vi "Clousure.vi"(8 "error in (no error)":errorcluster, 11 "CreatorA":refnum<class "CreatorA.lvclass">) -> (0 "error out":errorcluster, 3 "CreatorA":refnum<class "CreatorA.lvclass">)   [LabVIEW 2020, in "FactoryMethod.lvlib" / "FactoryMethodLazyEvaluation.lvlib" / "CreatorA.lvclass"]
uses:
  CreatorA.lvclass
  Creator/Creator.lvclass
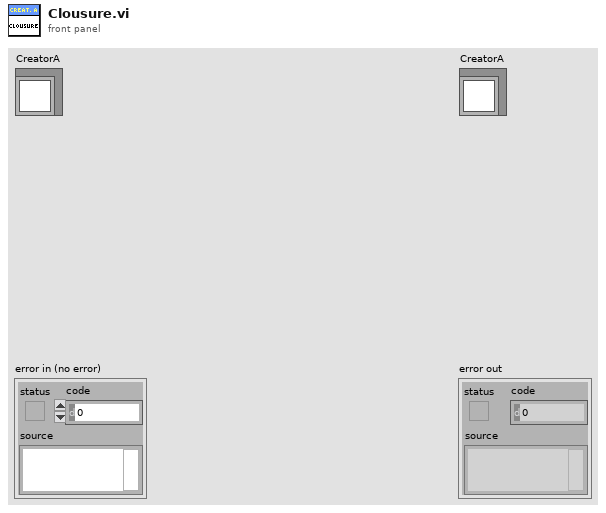
[diagram p1: front panel]
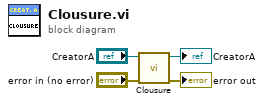
[diagram p0: block diagram]
diagram:
  n1 = call-parent "Clousure.vi"("error in (no error)"="error in (no error)", "Creator in"="CreatorA") -> ("error out"=→"error out":errorcluster, "Creator out"=→"CreatorA":refnum<class "CreatorA.lvclass">)  [unwired: 8 in]
